vi "getPanelRef.vi"(8 "error in (no error)":errorcluster, 11 "reference in":refnum<class "GUI Controller.lvclass">) -> (0 "error out":errorcluster, 2 "project_panels_ref":refnum<class "Project Panels.lvclass">, 3 "reference out":refnum<class "GUI Controller.lvclass">)   [LabVIEW 2016, in "GUI Controller.lvclass"]
uses:
  GUI Controller.lvclass
  Project Panels_class/Project Panels.lvclass
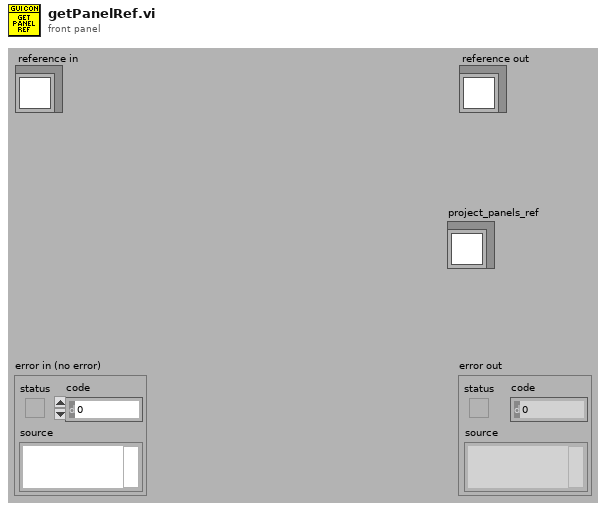
[diagram p1: front panel]
types:
  T1 = typedef "GUI Controller.lvclass/ObjectAttributesRef.ctl" = refnum<data-value>
  T2 = typedef "GUI Controller.lvclass/ObjectAttributes.ctl" = cluster{"MyAttribute":dbl, "state":T3, "project_panels_ref":refnum<class "Project Panels.lvclass">, "items_controller_ref":refnum<class "Items Controller.lvclass">, "notification_controller_ref":refnum<class "Notification Controller.lvclass">, "partstracking_controller_ref":refnum<class "PartsTracking Controller.lvclass">, "file_controller_ref":refnum<class "File Controller.lvclass">, "low_resolution?":bool, "run_python?":bool}
  T3 = typedef "GUI Controller.lvclass/state.ctl" = enum16{"initiate", "checkNotificationItems", "checkNotificationTracking", "operate", "updateFromFile", "stop"}
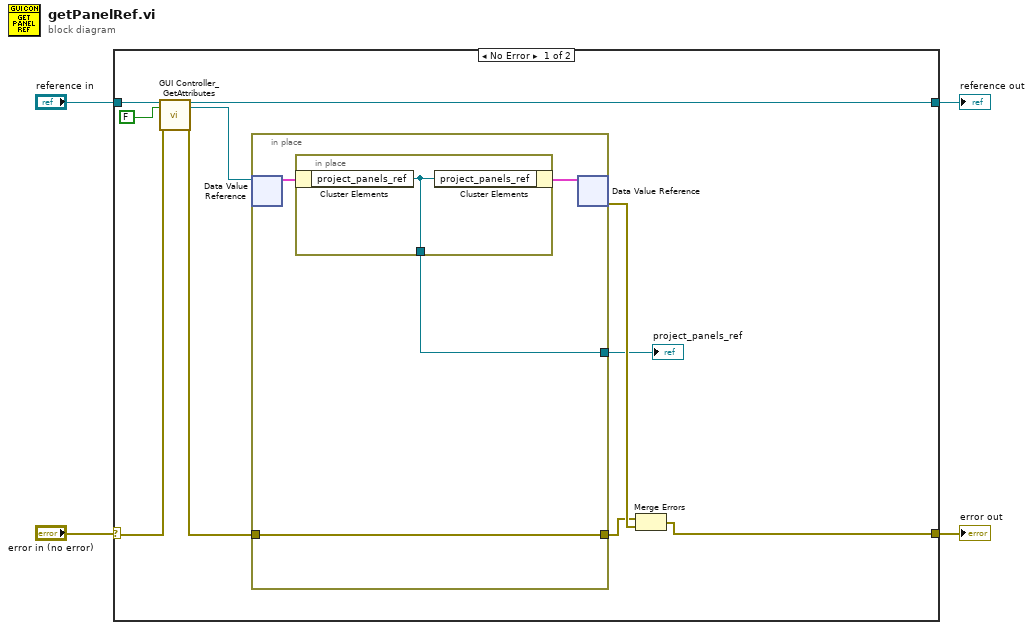
[diagram p0: block diagram]
diagram:
  n1 = case shown="No Error" "error in (no error)" {
    selector: "error in (no error)" -> [w9 w21]
    tunnel: [w14 w21] -> w3
    tunnel: [w7 w20] -> w1
    tunnel: "reference in" -> [w11 w20]
    frame No Error {
      n2 = call "GUI Controller_GetAttributes.vi"("reference in"=w11, "return data? (T)"=FALSE, "error in (no error)"=w9) -> ("reference out"=w7:refnum<class "GUI Controller.lvclass">, "attributes ref"=w6:T1, "error out"=w8:errorcluster)  [unwired: 13 in, 1 out]
      n3 = in-place {
        in-place-border: w8 -> [w16]
        in-place-border: [w16] -> w12
        in-place-border: [w15] -> w5
        n4 = in-place-dvr #1(w6) -> (w17:T2)  [unwired: 1 out]
        n5 = in-place {
          in-place-border: [w19] -> w15
          n6 = in-place-cluster #2(w17) -> ("project_panels_ref"=w19:refnum<class "Project Panels.lvclass">)
          n7 = in-place-cluster #2("project_panels_ref"=w19) -> (w18:T2)
        }
        n8 = in-place-dvr #1(w18) -> (w13:errorcluster)  [unwired: 1 out]
      }
      "project_panels_ref" <- w5
      n9 = Merge Errors(w12, w13) -> (w14:errorcluster)
    }
    frame Error {
    }
  }
  "error out" <- w3
  "reference out" <- w1
